vi "ReadCSV.vi"(8 "Error In":errorcluster caption="エラー入力", 9 "読み取り開始行":i32=1, 10 "行数(すべて:-1)":i32=-1, 11 "ファイルパス":path) -> (0 "Error Out":errorcluster caption="エラー出力", 3 "2D文字列":string[][](array[string]))   [LabVIEW 2014]
panel:
  out "EOF?":bool
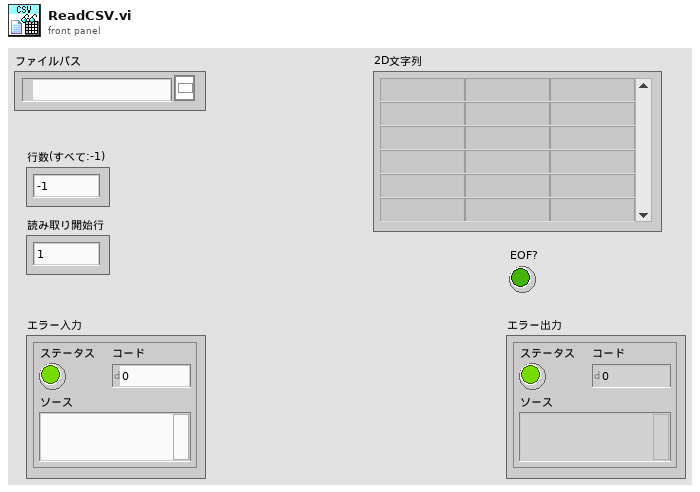
[diagram p1: front panel]
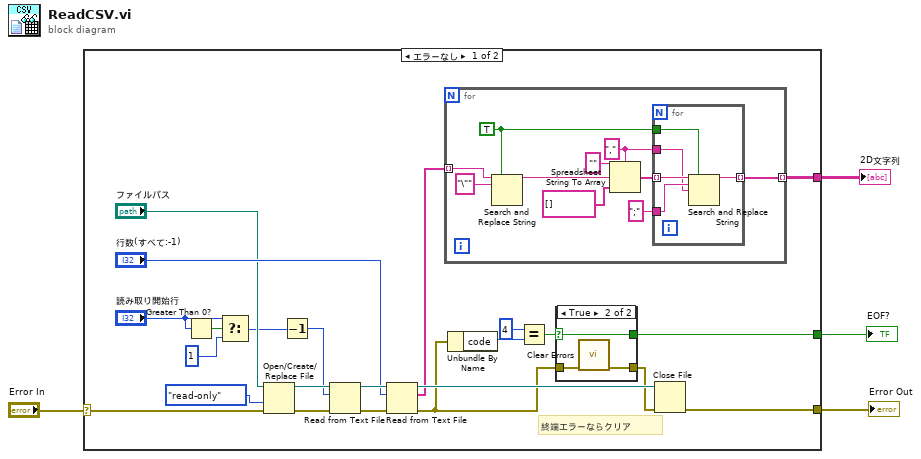
[diagram p0: block diagram]
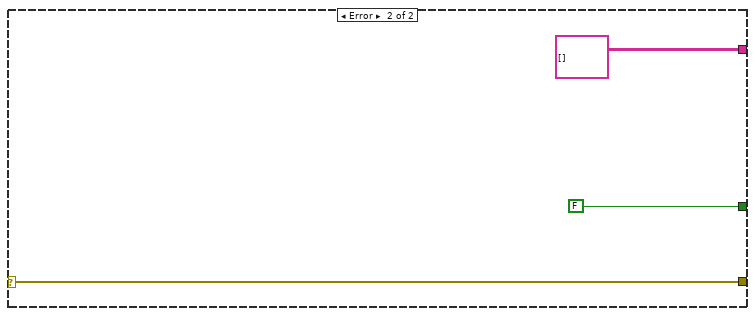
[diagram p3: hidden frame]
diagram:
  n1 = case shown="エラーなし" "Error In" {
    selector: "Error In" -> [w19 w49]
    tunnel: [w17 w49] -> w3
    tunnel: [w16 string[][] []] -> w2
    tunnel: [w6 FALSE] -> w1
    frame No Error {
      # "終端エラーならクリア"
      n2 = Greater Than 0?(x="読み取り開始行") -> (x > 0?=w15:bool)
      n3 = Select(t="読み取り開始行", s=w15, f=1) -> (s? t:f=w13:i32)
      n4 = Open/Create/Replace File(file path (use dialog)="ファイルパス", error in=w19, access (0:read/write)=enum16{"read/write", "read-only", "write-only"}."read-only" ("アクセス （0:read/write）")) -> (refnum out=w26:refnum<file>, error out=w25:errorcluster)  [unwired: 3 in, 1 out]
      n5 = Decrement(x=w13) -> (x-1=w18:i32)
      n6 = Read from Text File(file (use dialog)=w26, count=w18, error in=w25) -> (refnum out=w23:refnum<file>, error out=w24:errorcluster)  [unwired: 1 in, 2 out]
      n7 = Read from Text File(file (use dialog)=w23, count="行数(すべて:-1)", error in=w24) -> (refnum out=w27:refnum<file>, text=w5:string[], error out=w8:errorcluster)  [unwired: 1 in, 1 out]
      n8 = for {
        tunnel: w5 -> [w39] mode=indexing
        tunnel: [w35] -> w16 mode=indexing
        w36 = "," ("デリミタ（タブ）")
        w37 = TRUE ("すべて置換?（F）")
        n9 = Search and Replace String(replace all?=w37, input string=w39, search string="\"" ("検索文字列")) -> (result string=w33:string)  [unwired: 5 in, 3 out]
        n10 = Spreadsheet String To Array(delimiter (Tab)=w36, format string="" ("形式文字列"), spreadsheet string=w33, array type (2D Dbl)=string[] []) -> (array=w38:string[])
        n11 = for {
          tunnel: w38 -> [w47] mode=indexing
          tunnel: w37 -> [w46]
          tunnel: ";" ("置換文字列（\"\"）") -> [w45]
          tunnel: w36 -> [w44]
          tunnel: [w43] -> w35 mode=indexing
          n12 = Search and Replace String(replace all?=w46, input string=w47, search string=w45, replace string=w44) -> (result string=w43:string)  [unwired: 4 in, 3 out]
        }
      }
      n13 = Unbundle By Name(w8) -> ("code"=w11:i32)
      n14 = Equal?(x=4, y=w11) -> (x = y?=w9:bool)
      n15 = case shown="TRUE" w9 {
        selector: w9 -> [w28 w30]
        tunnel: w8 -> [w29 w32]
        tunnel: [w29 w31] -> w7
        tunnel: [w28 w30] -> w6
        frame False {
        }
        frame True {
          n16 = call <vilib>:"Clear Errors.vi"("error in (no error)"=w32) -> ("error out"=w31:errorcluster)  [unwired: 5 in, 1 out]
        }
      }
      n17 = Close File(refnum=w27, error in=w7) -> (error out=w17:errorcluster)  [unwired: 1 out]
    }
    frame Error {
    }
  }
  "Error Out" <- w3
  "2D文字列" <- w2
  "EOF?" <- w1
